vi "Parameterized.vi"() -> ()   [LabVIEW 2012]
doc: "This example inserts data into a table named parameterized in the LabVIEW.mdb database. The data is generated and inserted into the database once per second until you press the Stop button. \n\nThis VI uses a parameterized technique to insert data into the database. Since the SQL query can be parsed once and the data is \"filled in\" when needed, this results in a more efficient VI than if you used the Insert Data Into Database VI. However, the parameterized method is more difficult because it requires you to know more about SQL queries and data types."
uses:
  Auxilliary.llb/DB Tools Parameter Info.ctl
  Auxilliary.llb/DB Tools DataTypes.ctl
  Auxilliary.llb/DB Tools Parameter Dir.ctl
  Connection.llb/DB Tools Open Connec (Path).vi
  Command.llb/Cmd Delete.vi
  Auxilliary.llb/DB Tools Format Datetime String (Time Stamp).vi
  Command.llb/Cmd Set Parameter Value (C).vi
  Command.llb/Cmd Execute.vi
  Recordset.llb/Rec Destroy - Command.vi
  NI_Database_API_64.lvlib
panel:
  out "number of inserts":i32
  in  "stop":bool
  in  "parameters":T1[](array[typedef])=[{"parameter name"="DAQ channel", "type"=enum."String", "direction"=enum."Input", "value"=variant}, {"parameter name"="", "type"=enum."Date/Time", "direction"=enum."Input", "value"=variant}, {"parameter name"="data", "type"=enum."Binary", "direction"=enum."Input", "value"=variant}]
  # "notice that DAQ Channels are\nrepresented as strings in DB"
  # "parameter name is not required"
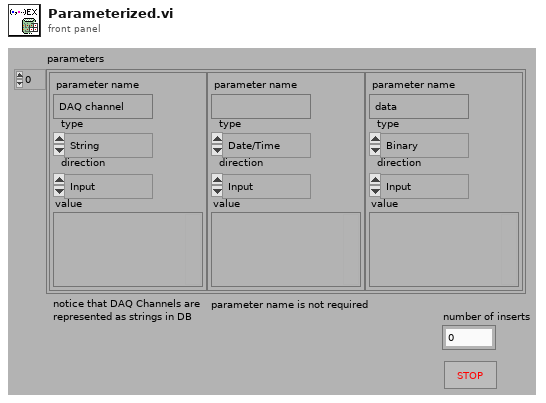
[diagram p1: front panel]
types:
  T1 = typedef "NI_Database_API_64.lvlib/DB Tools Parameter Info.ctl" = cluster{"parameter name":string, "type":T2, "direction":T3, "value":variant}
  T2 = typedef "NI_Database_API_64.lvlib/DB Tools DataTypes.ctl" = enum16{"String", "Long (I32)", "Single (SGL)", "Double (DBL)", "Date/Time", "Binary"}
  T3 = typedef "NI_Database_API_64.lvlib/DB Tools Parameter Dir.ctl" = enum32{"Input", "Output", "Input/Output", "Return Value"}
  T4 = typedef "NI_Database_API_64.lvlib/Conn ObjectReference.ctl" = refnum<k1>
  T5 = typedef "NI_Database_API_64.lvlib/Cmd ObjectReference.ctl" = refnum<k1>
  T6 = typedef "NI_Database_API_64.lvlib/Cmd-Rec Object Reference.ctl" = refnum<k1>
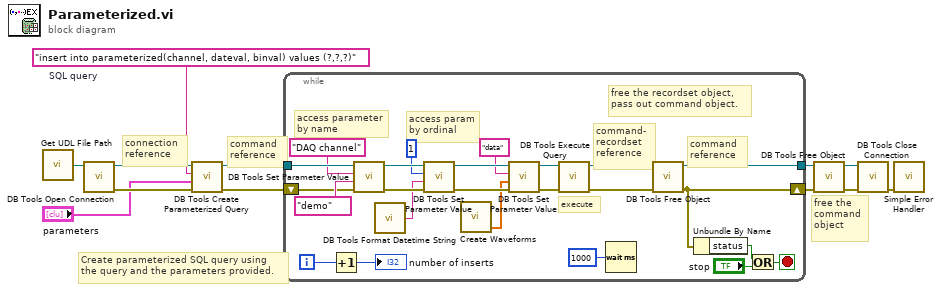
[diagram p0: block diagram]
diagram:
  w9 = "insert into parameterized(channel, dateval, binval) values (?,?,?)"  # SQL query
  # "command \nreference"
  # "free the\ncommand\nobject"
  # "connection \nreference"
  # "Create parameterized SQL query using \nthe query and the parameters provided."
  n1 = call "Get UDL File Path.vi"() -> ("UDL file path"=w1:path)  [unwired: 1 in]
  n2 = call-poly "DB Tools Open Connection.vi"("connection information"=w1) -> ("error out"=w12:errorcluster, "connection reference"=w11:T4)  [unwired: 7 in]
  n3 = call "DB Tools Create Parameterized Query.vi"("error in (no error)"=w12, "parameters"="parameters", "SQL query"=w9, "connection reference"=w11) -> ("error out"=w7:errorcluster, "command reference"=w10:T5)  [unwired: 3 in, 1 out]
  n4 = while {
    tunnel: w10 -> [w36]
    shift-right: [w22] -> w5
    shift-left: w7 -> [w26]
    tunnel: [w13] -> w6
    i -> [w18]
    stop <- w21 stop-if-true
    # "free the recordset object, \npass out command object."
    # "execute"
    # "command \nreference"
    # "command-\nrecordset \nreference"
    # "access param\nby ordinal"
    # "access parameter\nby name"
    n5 = Increment(x=w18) -> (x+1=→"number of inserts":i32)
    n6 = call-poly "DB Tools Set Parameter Value.vi"("error in (no error)"=w26, "value"=tag "demo", "parameter index"="DAQ channel", "command reference"=w36) -> ("error out"=w35:errorcluster, "command reference out"=w34:T5)  [unwired: 4 in]
    n7 = call-poly "DB Tools Format Datetime String.vi"() -> ("date/time string"=w29:string)  [unwired: 1 in]
    n8 = call-poly "DB Tools Set Parameter Value.vi"("error in (no error)"=w35, "value"=w29, "parameter index"=1, "command reference"=w34) -> ("error out"=w33:errorcluster, "command reference out"=w32:T5)  [unwired: 4 in]
    n9 = call "Create Waveforms.vi"() -> ("core temperature"=w15:dbl[])  [unwired: 3 in, 1 out]
    n10 = call-poly "DB Tools Set Parameter Value.vi"("error in (no error)"=w33, "value"=w15, "parameter index"="data", "command reference"=w32) -> ("error out"=w25:errorcluster, "command reference out"=w24:T5)  [unwired: 4 in]
    n11 = call-poly "DB Tools Execute Query.vi"("error in (no error)"=w25, "command reference"=w24) -> ("error out"=w23:errorcluster, "command-recordset reference"=w14:T6)  [unwired: 6 in]
    n12 = Wait (ms)(milliseconds to wait=u32 1000) -> ()  [unwired: 1 out]
    n13 = call-poly "DB Tools Free Object.vi"("error in (no error)"=w23, "command-recordset reference"=w14) -> ("error out"=w22:errorcluster, "command reference"=w13:T5)  [unwired: 8 in]
    n14 = Unbundle By Name(w22) -> ("status"=w19:bool)
    n15 = Or(x=w19, y="stop") -> (x .or. y?=w21:bool)
  }
  n16 = call-poly "DB Tools Free Object.vi"("error in (no error)"=w5, "command reference"=w6) -> ("error out"=w4:errorcluster, "connection reference"=w3:T4)  [unwired: 8 in]
  n17 = call "DB Tools Close Connection.vi"("error in (no error)"=w4, "connection reference"=w3) -> ("error out"=w2:errorcluster)  [unwired: 5 in]
  n18 = call <vilib>:"Simple Error Handler.vi"("error in (no error)"=w2) -> ()  [unwired: 4 in, 5 out]
